vi "Event_ball_inside_goalie_area.vi"(8 "error in (no error)":errorcluster, 10 "Game in":refnum<class "Game.lvclass">, 11 "Events in":refnum<class "Events.lvclass">) -> (0 "error out":errorcluster, 3 "Events out":refnum<class "Events.lvclass">)   [LabVIEW 2023, in "Events.lvclass"]
uses:
  Events.lvclass
  Game_class/Game.lvclass
  Game_class/Game.lvclass/Game.ctl
  Object_class/Object.lvclass/Object.ctl
  Parameters_class/Parameters.lvclass/Parameters.ctl
  Events.lvclass/Events.ctl
  Game_class/Read FieldRef.vi
  Game_class/Read BallRef.vi
  Game_class/Read Parameters.lvclass.vi
  Parameters_class/Read Area.vi
  Object_class/Read x.vi
  Object_class/Read y.vi
  Write ball_inside_our_goalie_area.vi
  Write ball_inside_enemy_goalie_area.vi
  Ball_class/Ball.lvclass
  Field_class/Field.lvclass
  Parameters_class/Parameters.lvclass
panel:
  out "Ball at goalkeeper area ?":bool
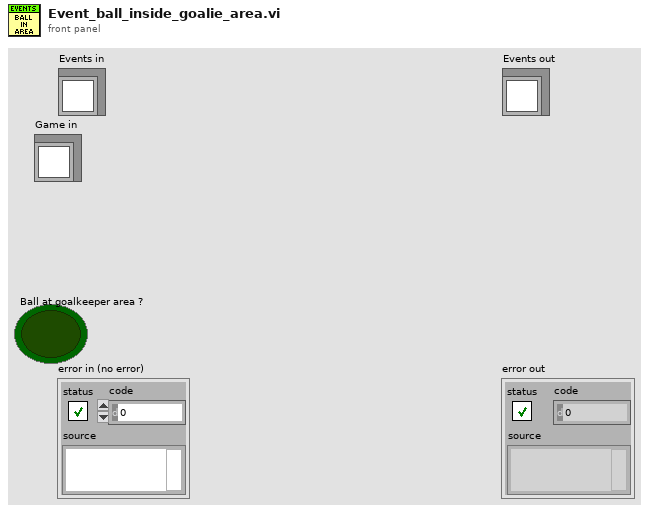
[diagram p1: front panel]
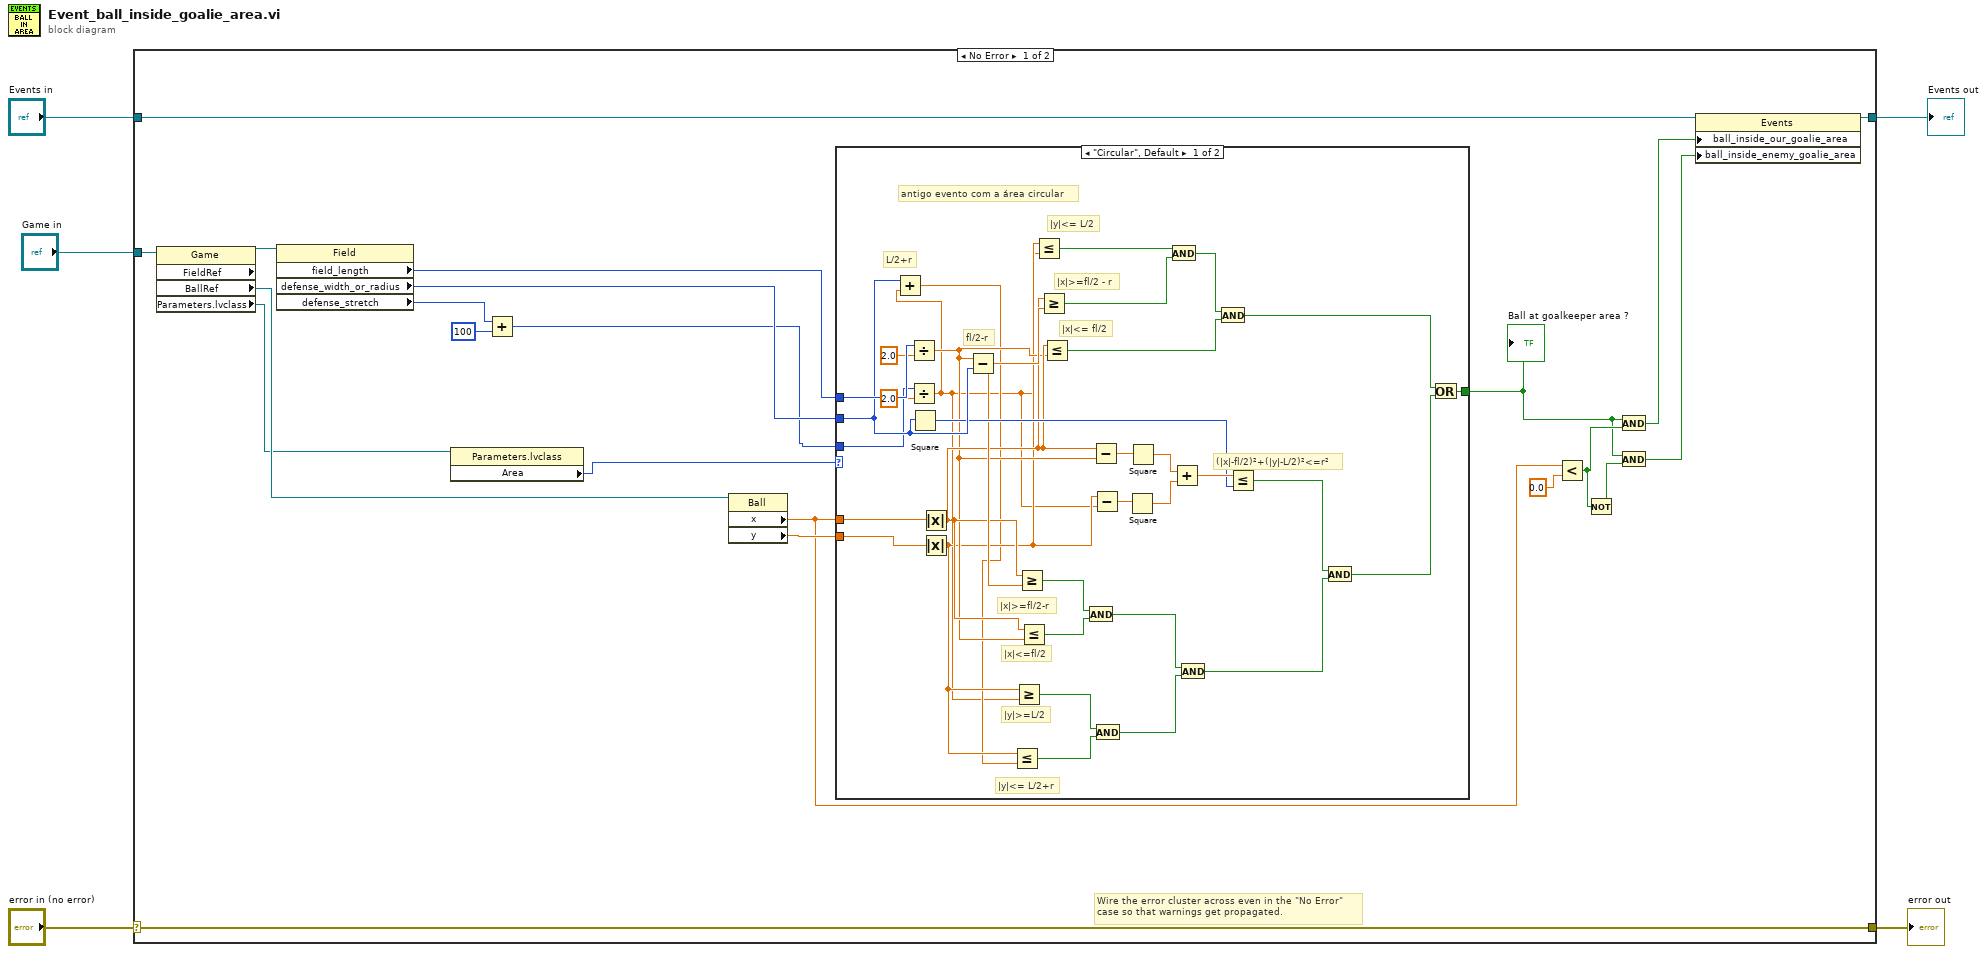
[diagram p0: block diagram]
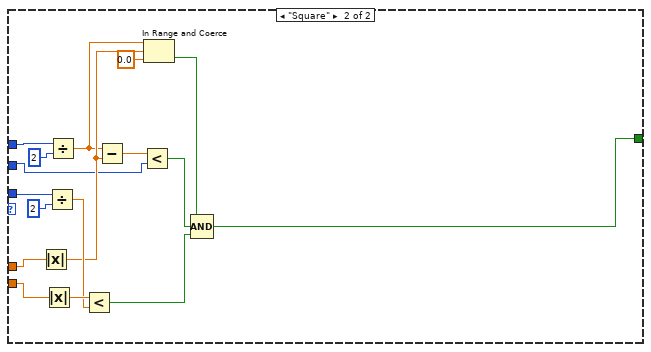
[diagram p2: hidden frame]
diagram:
  n1 = case shown="No Error" "error in (no error)" {
    selector: "error in (no error)" -> [w26 w79]
    tunnel: [w26 w79] -> w4
    tunnel: [w18 w78] -> w2
    tunnel: "Events in" -> [w19 w78]
    tunnel: "Game in" -> [w25 _]
    frame No Error {
      # "Wire the error cluster across even in the \"No Error\"\ncase so that warnings get propagated."
      n2 = property class="Game"(reference=w25) -> ("FieldRef"=w24:refnum<class "Field.lvclass">, "BallRef"=w21:refnum<class "Ball.lvclass">, "Parameters.lvclass"=w20:refnum<class "Parameters.lvclass">)  [unwired: 1 in, 2 out]
      n3 = property class="Field"(reference=w24) -> ("field_length"=w17:i32, "defense_width_or_radius"=w16:i32, "defense_stretch"=w22:i32)  [unwired: 1 in, 2 out]
      n4 = property class="Parameters.lvclass"(reference=w20) -> ("Area"=w14:enum16{"Circular", "Square"})  [unwired: 1 in, 2 out]
      n5 = Add(x=w22, y=u32 100) -> (x+y=w15:u32)
      n6 = property class="Ball"(reference=w21) -> ("x"=w12:dbl, "y"=w13:dbl)  [unwired: 1 in, 2 out]
      n7 = case shown="\"Circular\", Default" w14 {
        tunnel: w13 -> [w60 w65]
        tunnel: w12 -> [w59 w66]
        tunnel: w17 -> [w58 w63]
        tunnel: [w57 w61] -> w8
        tunnel: w16 -> [w56 w62]
        tunnel: w15 -> [w55 w64]
        frame "Circular", Default {
          # "antigo evento com a área circular"
          # "|y|<= L/2+r"
          # "L/2+r"
          # "|y|>=L/2"
          # "|x|<=fl/2"
          # "|x|>=fl/2-r"
          # "fl/2-r"
          # "(|x|-fl/2)²+(|y|-L/2)²<=r²"
          # "|x|<= fl/2"
          # "|x|>=fl/2 - r"
          # "|y|<= L/2"
          n8 = Divide(x=w58, y=2.0) -> (x/y=w38:dbl)
          n9 = Divide(x=w55, y=2.0) -> (x/y=w27:dbl)
          n10 = Add(x=w56, y=w27) -> (x+y=w36:dbl)
          n11 = Square(x=w56) -> (x^2=w43:i32)
          n12 = Absolute Value(x=w59) -> (abs(x)=w41:dbl)
          n13 = Absolute Value(x=w60) -> (abs(x)=w37:dbl)
          n14 = Subtract(x=w38, y=w56) -> (x-y=w42:dbl)
          n15 = Less Or Equal?(x=w37, y=w36) -> (x <= y?=w34:bool)
          n16 = Greater Or Equal?(x=w37, y=w27) -> (x >= y?=w35:bool)
          n17 = Greater Or Equal?(x=w41, y=w42) -> (x >= y?=w40:bool)
          n18 = Less Or Equal?(x=w41, y=w38) -> (x <= y?=w39:bool)
          n19 = Less Or Equal?(x=w37, y=w27) -> (x <= y?=w52:bool)
          n20 = Greater Or Equal?(x=w41, y=w42) -> (x >= y?=w51:bool)
          n21 = Less Or Equal?(x=w41, y=w38) -> (x <= y?=w49:bool)
          n22 = And(x=w40, y=w39) -> (x .and. y?=w33:bool)
          n23 = Subtract(x=w41, y=w38) -> (x-y=w48:dbl)
          n24 = Subtract(x=w37, y=w27) -> (x-y=w47:dbl)
          n25 = And(x=w35, y=w34) -> (x .and. y?=w32:bool)
          n26 = Square(x=w47) -> (x^2=w45:dbl)
          n27 = Square(x=w48) -> (x^2=w46:dbl)
          n28 = And(x=w52, y=w51) -> (x .and. y?=w50:bool)
          n29 = Add(x=w46, y=w45) -> (x+y=w44:dbl)
          n30 = And(x=w33, y=w32) -> (x .and. y?=w30:bool)
          n31 = And(x=w50, y=w49) -> (x .and. y?=w29:bool)
          n32 = Less Or Equal?(x=w44, y=w43) -> (x <= y?=w31:bool)
          n33 = And(x=w31, y=w30) -> (x .and. y?=w28:bool)
          n34 = Or(x=w29, y=w28) -> (x .or. y?=w57:bool)
        }
        frame "Square" {
          n35 = Absolute Value(x=w66) -> (abs(x)=w70:dbl)
          n36 = Absolute Value(x=w65) -> (abs(x)=w76:dbl)
          n37 = Divide(x=w64, y=u32 2) -> (x/y=w73:dbl)
          n38 = Divide(x=w63, y=u32 2) -> (x/y=w68:dbl)
          n39 = Less?(x=w76, y=w73) -> (x < y?=w71:bool)
          n40 = Subtract(x=w68, y=w70) -> (x-y=w75:dbl)
          n41 = Less?(x=w75, y=w62) -> (x < y?=w72:bool)
          n42 = In Range and Coerce(upper limit=w68, x=w70, lower limit=0.0) -> (In Range?=w67:bool)  [unwired: 1 out]
          n43 = Compound Arithmetic op=AND(w67, w72, w71) -> (w61:bool)
        }
      }
      "Ball at goalkeeper area ?" <- w8
      n44 = Less?(x=w12, y=0.0) -> (x < y?=w9:bool)
      n45 = Not(x=w9) -> (.not. x?=w10:bool)
      n46 = And(x=w8, y=w9) -> (x .and. y?=w7:bool)
      n47 = And(x=w8, y=w10) -> (x .and. y?=w6:bool)
      n48 = property class="Events"(reference=w19, "ball_inside_our_goalie_area"=w7, "ball_inside_enemy_goalie_area"=w6) -> (reference out=w18:refnum<class "Events.lvclass">)  [unwired: 1 in, 1 out]
    }
    frame Error {
    }
  }
  "error out" <- w4
  "Events out" <- w2
